vi "Global 1.vi"() -> ()   [LabVIEW 2013]
panel:
  in  "Packets":cluster{"t0":dbl, "dt":dbl, "Y":cdb[]}[](array[cluster])
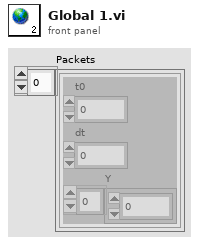
[diagram p1: front panel]
diagram:
